vi "15- Addition of 2 input strings(SubVI).vi"(10 "Input string 2":string, 11 "Input string 1":string) -> (3 "Output string":string)   [LabVIEW 2019]
panel:
  # "SUBVI for addition of 2 input strings"
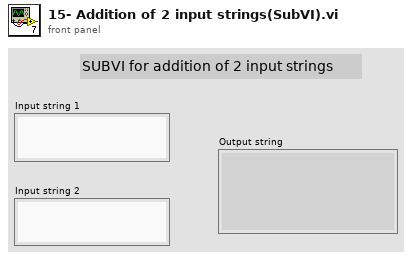
[diagram p1: front panel]
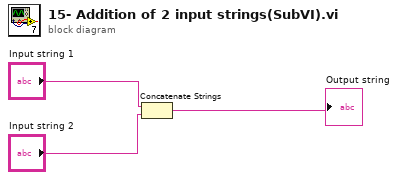
[diagram p0: block diagram]
diagram:
  n1 = Concatenate Strings("Input string 1", "Input string 2") -> (→"Output string":string)
